vi "yforcetestnodrag.vi"() -> (3 "function return":dbl)   [LabVIEW 2017, in "HapticSTM.lvlib"]
doc: "extern \"C\" __declspec(dllexport) double yforcetestnodrag();"
uses:
  <userlib>/HapticSTM/Feedbackless - Testdata/Project/HapticSTM.lvlib
  <userlib>/HapticSTM/HapticSTM.dll
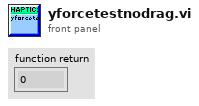
[diagram p1: front panel]
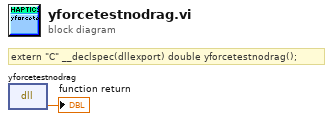
[diagram p0: block diagram]
diagram:
  # "extern \"C\" __declspec(dllexport) double yforcetestnodrag();"
  n1 = dll-call lib="C:/Program Files/National Instruments/LabVIEW 2019/user.lib/HapticSTM/HapticSTM.*" fn="yforcetestnodrag"() -> (→"function return":dbl)  [unwired: 3 in, 2 out]
